vi "Digital_IO_Example.vi"() -> ()   [LabVIEW 2021]
uses:
  <vilib>/Galil/resources/gclib/gclib.lvlib
panel:
  out "DO 1 Status":string
  out "DI Bank 0 Bitmask":string
  in  "stop":bool
  in  "OP":u16=85
  in  "IP Address":string="192.168.1.77"
  out "error out":errorcluster
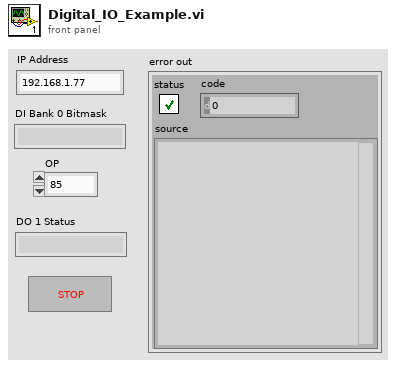
[diagram p1: front panel]
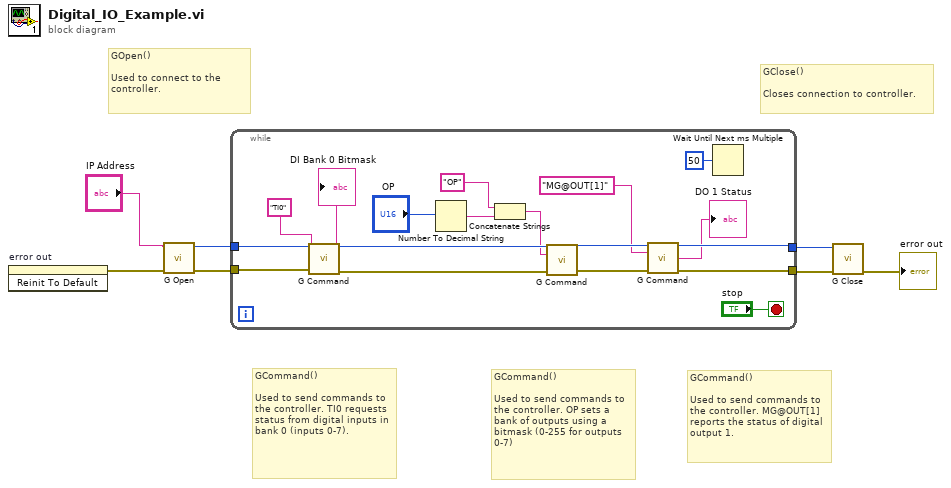
[diagram p0: block diagram]
diagram:
  # "GCommand()\n\nUsed to send commands to the controller. MG@OUT[1] reports the status of digital output 1."
  # "GCommand()\n\nUsed to send commands to the controller. OP sets a bank of outputs using a bitmask (0-255 for outputs 0-7)"
  # "GCommand()\n\nUsed to send commands to the controller. TI0 requests status from digital inputs in bank 0 (inputs 0-7)."
  # "GClose()\n\nCloses connection to controller."
  # "GOpen()\n\nUsed to connect to the controller."
  n1 = invoke on="error out" class="Clust (strict)" method="Reinit To Default"() -> (error out=w5:errorcluster)  [unwired: 3 in, 2 out]
  n2 = call <vilib>:"G Open.vi"("error in (no error)"=w5, "address"="IP Address") -> ("error out"=w4:errorcluster, "g out"=w7:u64)  [unwired: 7 in]
  n3 = while {
    tunnel: w4 -> [w15]
    tunnel: w7 -> [w14]
    tunnel: [w9] -> w3
    tunnel: [w10] -> w1
    stop <- "stop" stop-if-true
    n4 = call <vilib>:"G Command.vi"("g"=w14, "command"="TI0" ("buffer"), "error in (no error)"=w15) -> ("g out"=w20:u64, "buffer out"=→"DI Bank 0 Bitmask":string, "error out"=w16:errorcluster)  [unwired: 10 in]
    n5 = Number To Decimal String(number="OP") -> (decimal integer string=w18:string)  [unwired: 1 in]
    n6 = Concatenate Strings("OP" ("string"), w18) -> (w17:string)
    n7 = call <vilib>:"G Command.vi"("g"=w20, "command"=w17, "error in (no error)"=w16) -> ("g out"=w13:u64, "error out"=w11:errorcluster)  [unwired: 10 in, 1 out]
    n8 = call <vilib>:"G Command.vi"("g"=w13, "command"="MG@OUT[1]", "error in (no error)"=w11) -> ("g out"=w9:u64, "buffer out"=→"DO 1 Status":string, "error out"=w10:errorcluster)  [unwired: 10 in]
    n9 = Wait Until Next ms Multiple(millisecond multiple=u32 50) -> ()  [unwired: 1 out]
  }
  n10 = call <vilib>:"G Close.vi"("error in (no error)"=w1, "g"=w3) -> ("error out"=→"error out":errorcluster)  [unwired: 9 in]
